vi "Parse Response JSON.vi"(8 "error in (no error)":errorcluster, 10 "Response JSON":string, 11 "RGetSceneItemEnabled in":refnum<class "RGetSceneItemEnabled.lvclass">) -> (0 "error out":errorcluster, 3 "RGetSceneItemEnabled out":refnum<class "RGetSceneItemEnabled.lvclass">)   [LabVIEW 2022 SP3, in "obs-websocket-lv.lvlib" / "RGetSceneItemEnabled.lvclass"]
uses:
  RGetSceneItemEnabled.lvclass
  RGetSceneItemEnabled.lvclass/RGetSceneItemEnabled.ctl
  <vilib>/IlluminatedG/lv-web-crypto/lv-json/JSON/JSON.lvlib
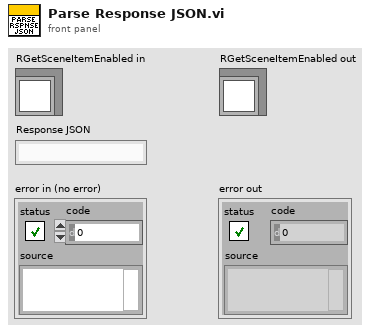
[diagram p1: front panel]
types:
  T1 = typedef "JSON.lvlib/JSON Item Type.ctl" = enum16{"unknown", "null", "Array", "Object", "String", "Number", "Boolean"}
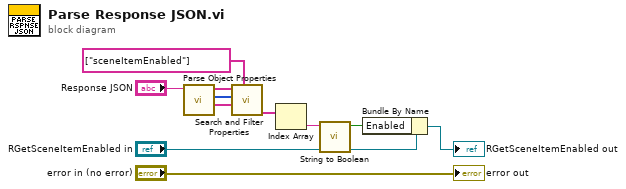
[diagram p0: block diagram]
diagram:
  n1 = call <vilib>:"Parse Object Properties.vi"("JSON String"="Response JSON") -> ("Values"=w6:string[], "Item Types"=w7:T1[], "Keys"=w8:string[])  [unwired: 7 in, 1 out]
  n2 = call <vilib>:"Search and Filter Properties.vi"("Search Keys"=string[] ["sceneItemEnabled"], "Values In"=w6, "Types In"=w7, "Keys In"=w8) -> ("Filtered Values"=w4:string[])  [unwired: 2 in, 5 out]
  n3 = Index Array(array=w4) -> (element=w3:string)  [unwired: 1 in]
  n4 = call <vilib>:"String to Boolean.vi"("Bool String"=w3) -> ("Boolean"=w1:bool)  [unwired: 10 in]
  n5 = Bundle By Name(cluster="RGetSceneItemEnabled in", "Enabled"=w1) -> (→"RGetSceneItemEnabled out":refnum<class "RGetSceneItemEnabled.lvclass">)
  "error out" <- "error in (no error)"
